vi "信息转换.vi"(7 "联机模式":enum16{"单机", "追溯"}(ring)=enum."追溯", 8 "错误输入（无错误）":errorcluster, 10 "追溯码":string[](array[string]), 11 "测试信息":T1) -> (0 "错误输出":errorcluster, 3 "信息输出":string[](array[string]))   [LabVIEW 2020]
panel:
  # "用户信息转换"
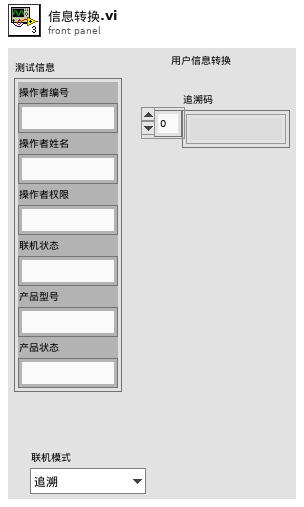
[diagram p1: front panel]
types:
  T1 = cluster{"操作者编号":string, "操作者姓名":string, "操作者权限":string, "联机状态":string, "产品型号":string, "产品状态":string}
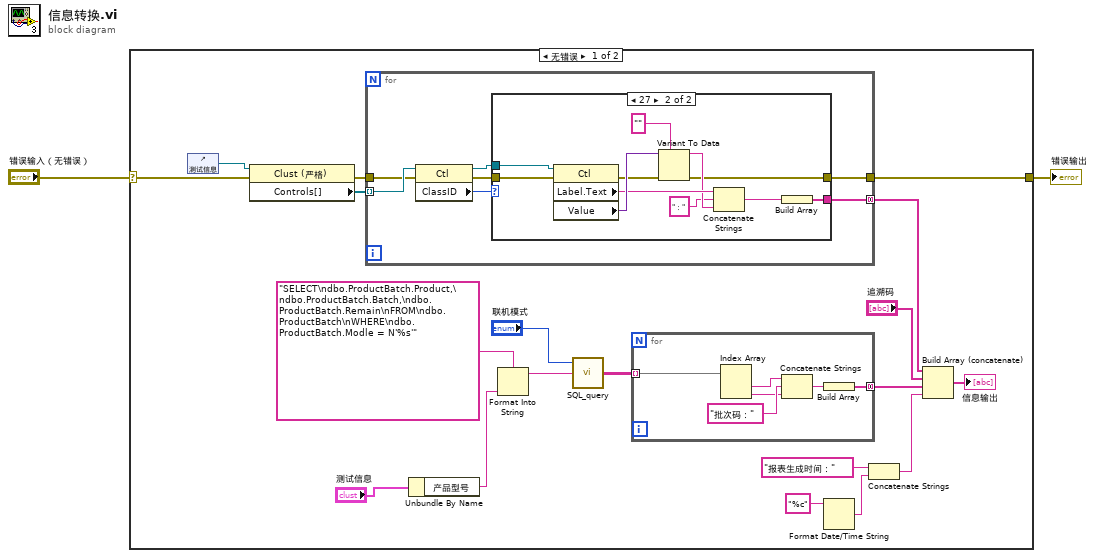
[diagram p0: block diagram]
diagram:
  n1 = case shown="无错误" "错误输入（无错误）" {
    selector: "错误输入（无错误）" -> [w14 w47]
    tunnel: [w12 w47] -> w1
    frame No Error {
      n2 = control-ref of="测试信息"() -> (w21:refnum<vi>)
      n3 = property on="属性节点" class="Clust (严格)"(reference=w21, error in=w14) -> (error out=w13:errorcluster, "Controls[]"=w20:refnum<vi>[])  [unwired: 1 out]
      n4 = for {
        tunnel: w20 -> [w34] mode=indexing
        tunnel: [w31] -> w18 mode=concatenating
        tunnel: w13 -> [w30]
        tunnel: [w28] -> w12
        n5 = property class="Ctl"(reference=w34, error in=w30) -> (reference out=w32:refnum<vi>, error out=w29:errorcluster, "ClassID"=w33:u32)
        n6 = case shown="27" w33 {
          tunnel: w32 -> [_ w46]
          tunnel: [_ w39] -> w31
          tunnel: w29 -> [w35 w38]
          tunnel: [w35 w36] -> w28
          frame 0, Default {
          }
          frame 27 {
            n7 = property class="Ctl"(reference=w46, error in=w38) -> (error out=w37:errorcluster, "Label.Text"=w43:string, "Value"=w44:variant)  [unwired: 1 out]
            n8 = Variant To Data(error in=w37, type="", Variant=w44) -> (data=w42:string, error out=w36:errorcluster)
            n9 = Concatenate Strings(w43, "：" ("字符串"), w42) -> (w40:string)
            n10 = Build Array(w40) -> (w39:string[])
          }
        }
      }
      n11 = Unbundle By Name("测试信息") -> ("产品型号"=w7:string)
      n12 = Format Into String(format string="SELECT\ndbo.ProductBatch.Product,\ndbo.ProductBatch.Batch,\ndbo.ProductBatch.Remain\nFROM\ndbo.ProductBatch\nWHERE\ndbo.ProductBatch.Modle = N'%s'" ("SQL query"), w7) -> (resulting string=w6:string)  [unwired: 2 in, 1 out]
      n13 = call "SQL_query.vi"("SQL query"=w6, "联机模式"="联机模式") -> ("data"=w5:string[][])  [unwired: 2 in, 1 out]
      n14 = for {
        tunnel: w5 -> [w25] mode=indexing
        tunnel: [w22] -> w10 mode=concatenating
        n15 = Index Array(array=w25) -> (element #1=w24:string, element #2=w23:string)  [unwired: 2 in]
        n16 = Concatenate Strings(w24, "批次码：" ("字符串"), w23) -> (w26:string)
        n17 = Build Array(w26) -> (w22:string[])
      }
      n18 = Format Date/Time String(time format string (%c)="%c") -> (date/time string=w15:string)  [unwired: 2 in]
      n19 = Concatenate Strings("报表生成时间：" ("字符串"), w15) -> (w9:string)
      n20 = Build Array (concatenate)(w18, "追溯码", w10, w9) -> (→"信息输出":string[])
    }
    frame Error {
    }
  }
  "错误输出" <- w1
